vi "Configure Pulse Power.vi"(8 "error in (no error)":errorcluster, 9 "Duty Cycle (1 %)":dbl=1.0, 10 "Enable Pulse Power (T: Enable)":bool=TRUE, 11 "VISA resource name":refnum<visa-resource-name>) -> (0 "error out":errorcluster, 3 "VISA resource name out":refnum<visa-resource-name>)   [LabVIEW 2018, in "Agilent U2000 Series.lvlib"]
doc: "Enables or disables the pulse power measurement and set the duty cycle for the pulse power measurement.\n\nNote: \nThis VI is only applicable for U2040 X-Series."
uses:
  Agilent U2000 Series.lvlib
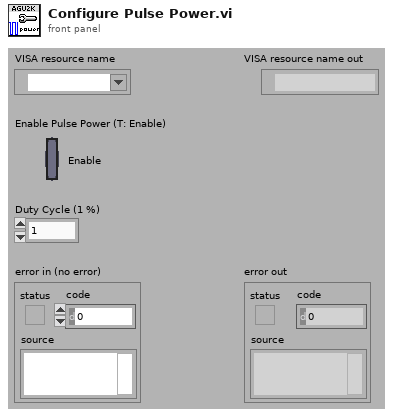
[diagram p1: front panel]
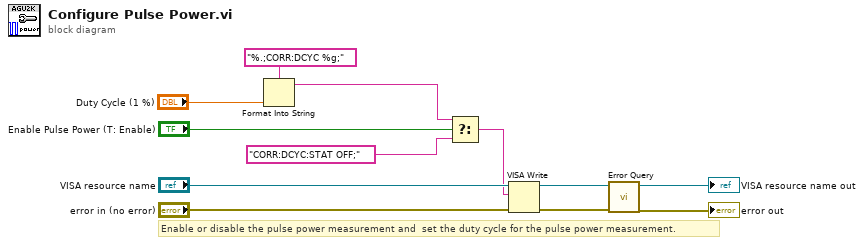
[diagram p0: block diagram]
diagram:
  # "Enable or disable the pulse power measurement and  set the duty cycle for the pulse power measurement."
  n1 = Format Into String(format string="%.;CORR:DCYC %g;", "Duty Cycle (1 %)") -> (resulting string=w2:string)  [unwired: 2 in, 1 out]
  n2 = Select(t=w2, s="Enable Pulse Power (T: Enable)", f="CORR:DCYC:STAT OFF;") -> (s? t:f=w3:string)
  n3 = VISA Write(VISA resource name="VISA resource name", write buffer=w3, error in (no error)="error in (no error)") -> (VISA resource name out=w8:refnum<visa-resource-name>, error out=w7:errorcluster)  [unwired: 1 out]
  n4 = call "Error Query.vi"("error in (no error)"=w7, "VISA resource name"=w8) -> ("error out"=→"error out":errorcluster, "VISA resource name out"=→"VISA resource name out":refnum<visa-resource-name>)  [unwired: 6 in, 2 out]
